vi "Add.vi"(8 "error in (no error)":errorcluster, 10 "BC ID":i32, 11 "BCReg":refnum<data-value>) -> (0 "error out":errorcluster, 2 "First?":bool, 3 "BCReg":refnum<data-value>)   [LabVIEW 2017, in "BusController.lvlib" / "BCReg.lvclass"]
uses:
  BCReg.lvclass
  BCReg.lvclass/BCReg.ctl
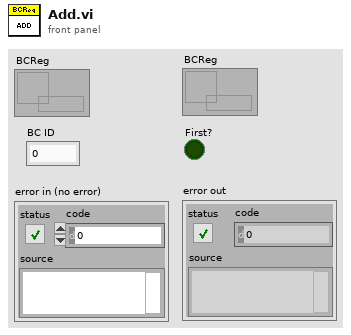
[diagram p1: front panel]
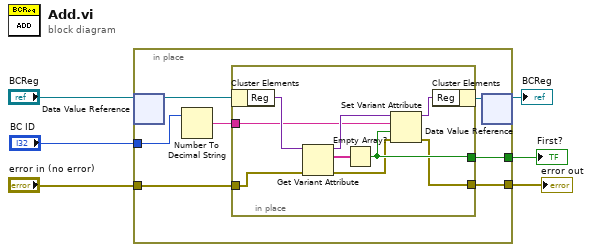
[diagram p0: block diagram]
diagram:
  n1 = in-place {
    in-place-border: "BC ID" -> [w13]
    in-place-border: "error in (no error)" -> [w10]
    in-place-border: [w8] -> w2
    in-place-border: [w7] -> w3
    n2 = in-place-dvr #1("BCReg") -> (w12:refnum<class "BCReg.lvclass">)  [unwired: 1 out]
    n3 = Number To Decimal String(number=w13) -> (decimal integer string=w11:string)  [unwired: 1 in]
    n4 = in-place {
      in-place-border: w11 -> [w19]
      in-place-border: w10 -> [w18]
      in-place-border: [w16] -> w8
      in-place-border: [w14] -> w7
      n5 = in-place-cluster #2(w12) -> ("Reg"=w22:variant)
      n6 = Get Variant Attribute(Variant=w22, error in=w18) -> (duplicate Variant=w20:variant, names=w21:string[], error out=w15:errorcluster)  [unwired: 2 in, 1 out]
      n7 = Empty Array?(array=w21) -> (empty?=w16:bool)
      n8 = Set Variant Attribute(Variant=w20, name=w19, value=w16, error in=w15) -> (Variant out=w17:variant, error out=w14:errorcluster)  [unwired: 1 out]
      n9 = in-place-cluster #2("Reg"=w17) -> (w9:refnum<class "BCReg.lvclass">)
    }
    n10 = in-place-dvr #1(w9) -> (→"BCReg":refnum<data-value>)  [unwired: 1 out]
  }
  "error out" <- w3
  "First?" <- w2
